vi "clusterDataChecking.vi"(0 "Cluster input":cluster{"Numeric 2":dbl, dbl}) -> (1 "value output":dbl, 2 "index output":i32, 3 "Array":cluster{"Numeric 2":dbl, dbl}[](array[cluster]))   [LabVIEW 2017]
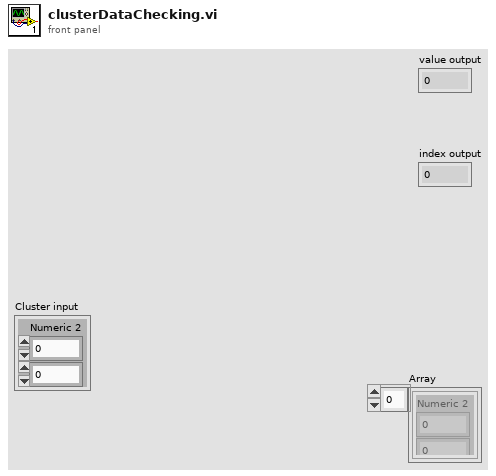
[diagram p1: front panel]
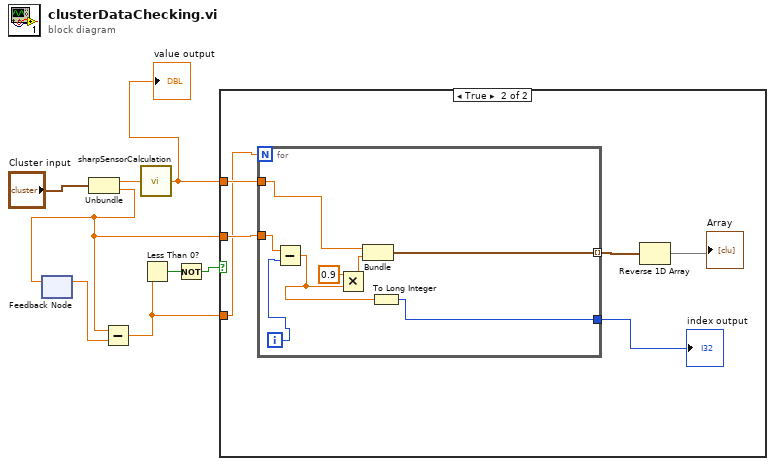
[diagram p0: block diagram]
diagram:
  n1 = feedback #1() -> (w4:dbl)  [unwired: 1 in]
  n2 = Unbundle("Cluster input") -> ("Numeric 2"=w8:dbl, w6:dbl)
  n3 = feedback-in #1(w6) -> ()
  n4 = Subtract(x=w6, y=w4) -> (x-y=w3:dbl)
  n5 = call "sharpSensorCalculation.vi"("y"=w8) -> ("Numeric 2"=w5:dbl)
  "value output" <- w5
  n6 = Less Than 0?(x=w3) -> (x < 0?=w2:bool)
  n7 = Not(x=w2) -> (.not. x?=w1:bool)
  n8 = case shown="True" w1 {
    tunnel: w6 -> [_ w14]
    tunnel: w5 -> [_ w13]
    tunnel: w3 -> [_ w11]
    frame False {
    }
    frame True {
      n9 = for {
        N: w11 -> [_]
        tunnel: w14 -> [w19]
        tunnel: w13 -> [w20]
        tunnel: [w16] -> w12
        tunnel: [w15] -> w10 mode=indexing
        i -> [w18]
        n10 = Subtract(x=w19, y=w18) -> (x-y=w17:dbl)
        n11 = Multiply(x=0.9, y=w17) -> (x*y=w22:dbl)
        n12 = Bundle("Numeric 2"=w20, w22) -> (w15:cluster{"Numeric 2":dbl, dbl})  [unwired: 1 in]
        n13 = To Long Integer(number=w17) -> (32bit integer=w16:i32)
      }
      "index output" <- w12
      n14 = Reverse 1D Array(array=w10) -> (reversed array=→"Array":cluster{"Numeric 2":dbl, dbl}[])
    }
  }
